vi "自动升级更新main.vi"() -> ()   [LabVIEW 2016, in "自动更新.lvlib"]
panel:
  out "waittime":u8
  out "有新版本":bool
  out "下载的文件名":string
  out "最新版本获取进度":u8(slide) scale=0.0..100.0
  # "版本获取中，请稍后！"
  # "s"
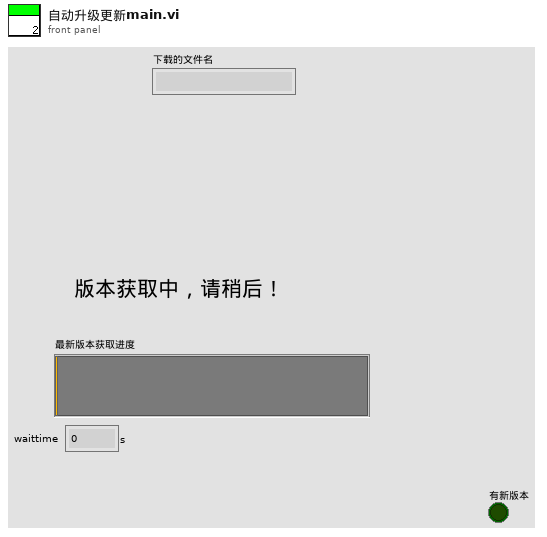
[diagram p1: front panel]
types:
  T1 = enum16{"get version information", "get success", "contact", "over"}
  T2 = cluster{"网络灯":bool, "接收中":bool, "已接收百分比":u8, "接收成功次数":dbl, "当前步骤":enum16{"init", "receivehead", "receivecontent", "receivesuccess", "over"}, "文件名":string, "error out":errorcluster}
  T3 = enum16{"open", "replace", "create", "open or create", "replace or create", "replace or create with confirmation"}
  T4 = enum32{"Bad", "Idle", "Run top level", "Running"}
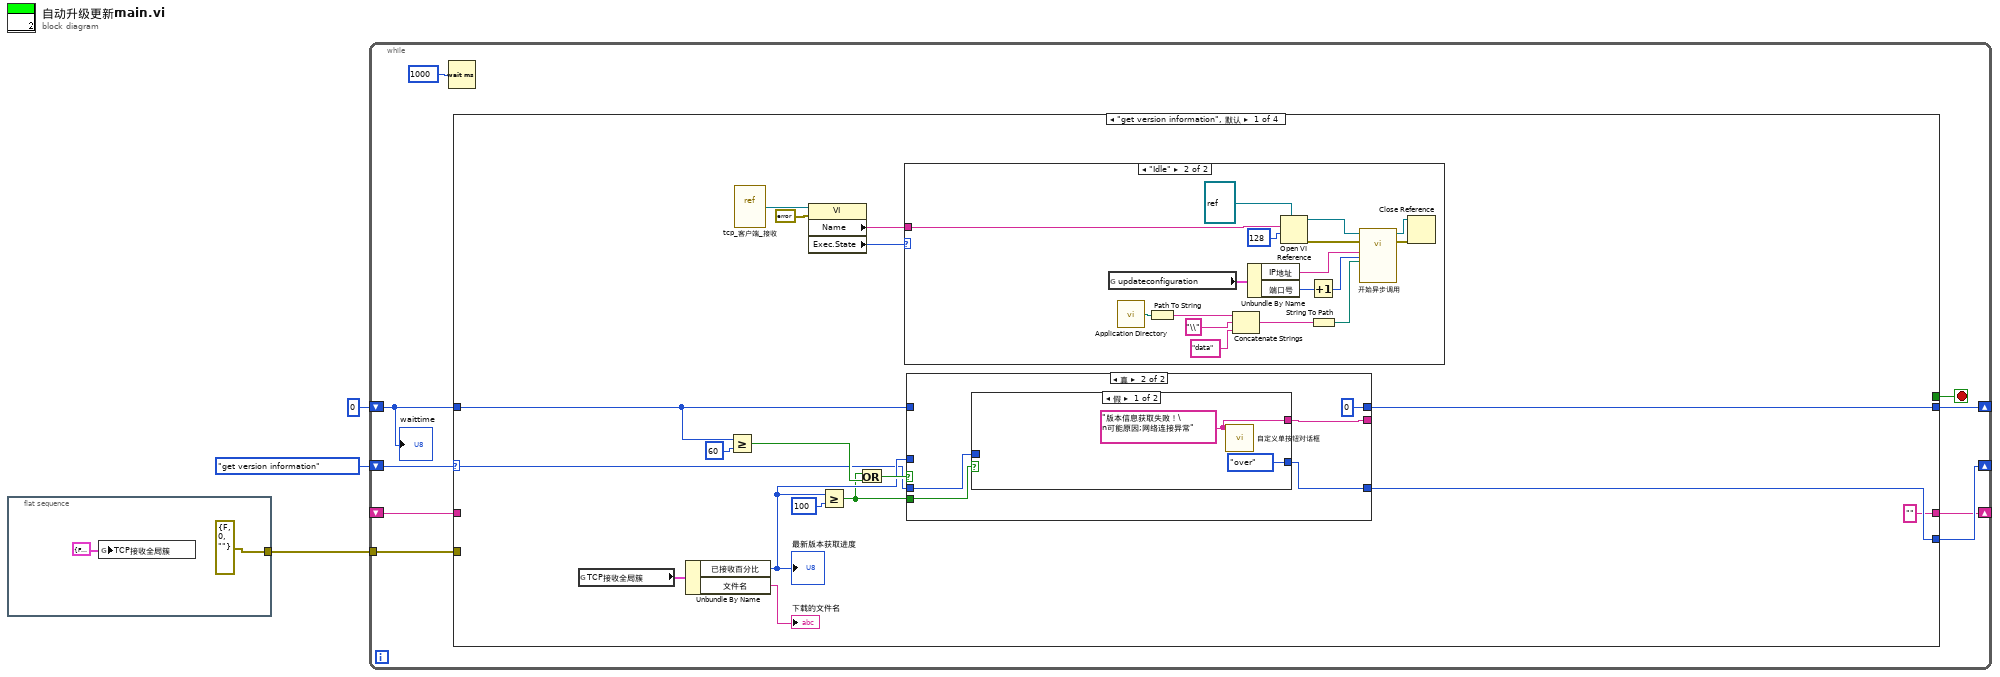
[diagram p0: block diagram]
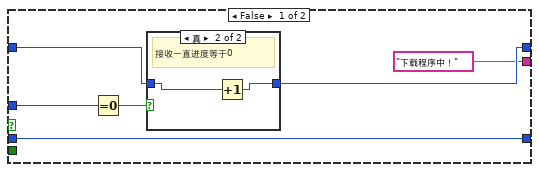
[diagram p2: hidden frame]
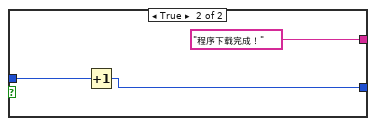
[diagram p4: hidden frame]
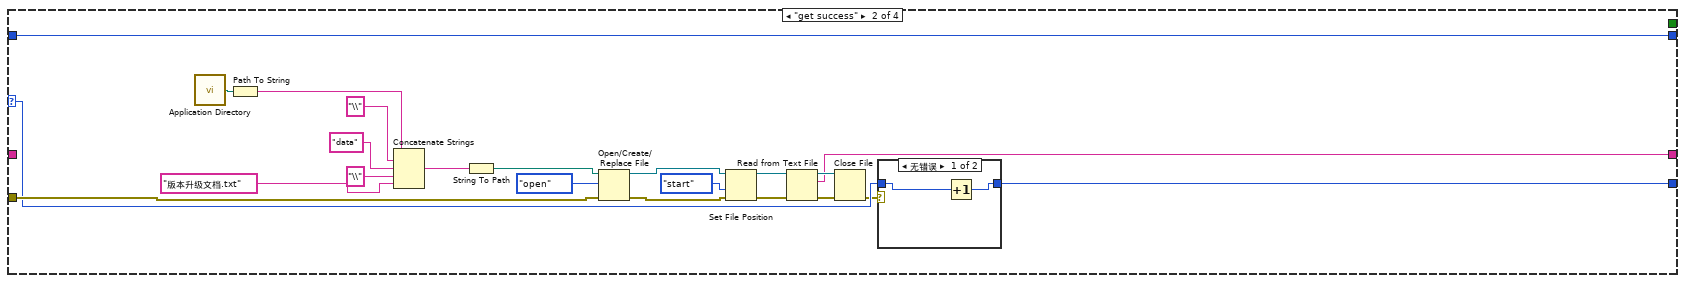
[diagram p6: hidden frame]
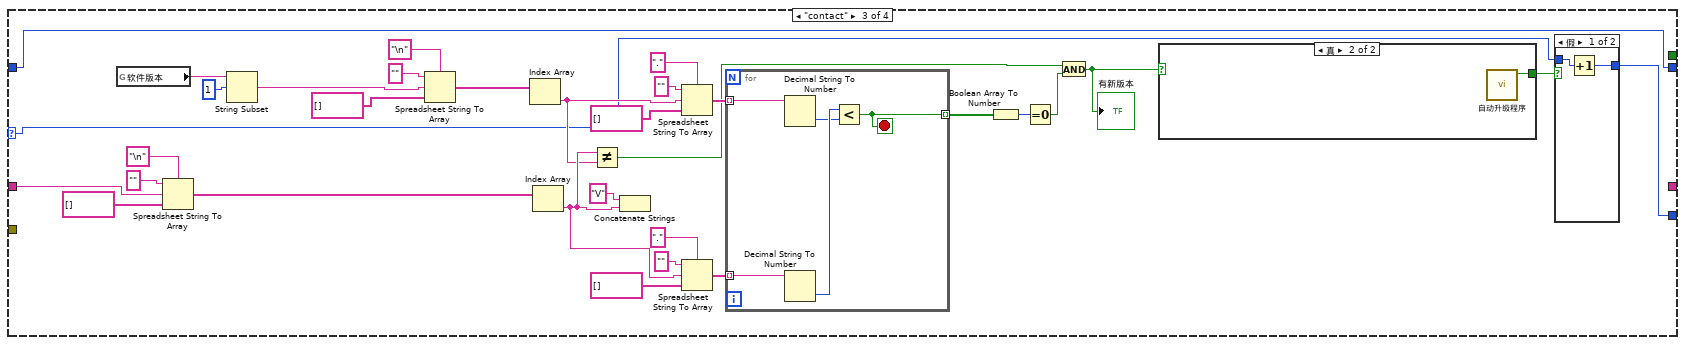
[diagram p8: hidden frame]
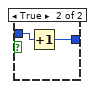
[diagram p9: hidden frame]
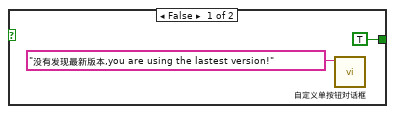
[diagram p10: hidden frame]
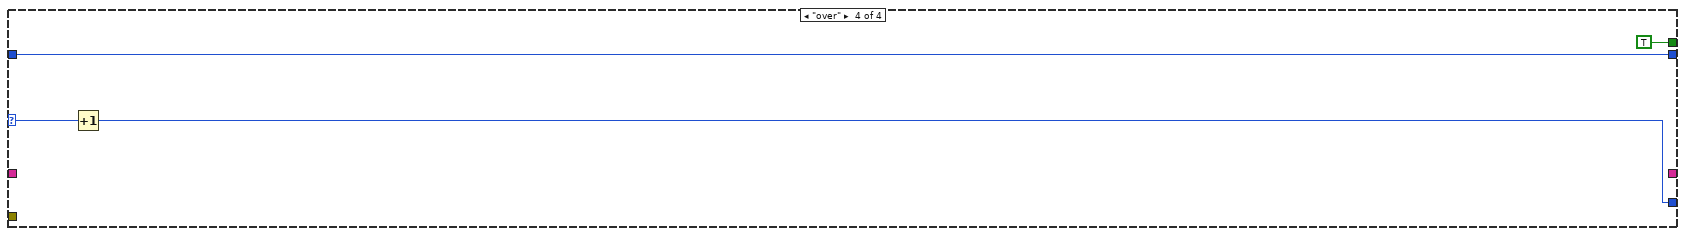
[diagram p11: hidden frame]
diagram:
  n1 = flat-sequence {
    tunnel: [errorcluster {"status"=FALSE, "code"=0, "source"=""} ("错误常量")] -> w1
    frame #0 {
      n2 = global write "全局变量1.vi" "TCP接收全局簇"(T2 {"网络灯"=FALSE, "接收中"=FALSE, "已接收百分比"=0, "接收成功次数"=0.0, "当前步骤"=enum."init", "文件名"="", "error out"={"status"=FALSE, "code"=0, "source"=""}} ("TCP接收全局簇")) -> ()
    }
  }
  n3 = while {
    shift-right: [w10] -> _
    shift-left: T1."get version information" -> [w13]
    shift-right: [w11] -> _
    shift-left: u8 0 ("y") -> [w12]
    tunnel: w1 -> [w9]
    shift-right: [w8] -> _
    shift-left: _ -> [w7]
    stop <- w6 stop-if-true
    n4 = Wait (ms)(milliseconds to wait=u32 1000 ("等待时间（毫秒）")) -> ()  [unwired: 1 out]
    n5 = case shown="\"get version information\", 默认" w13 {
      selector: w13 -> [w17 w76 w95 w138]
      tunnel: w12 -> [w19 w68 w93 w139]
      tunnel: [w18 w68 w93 w139] -> w11
      tunnel: [w16 w75 w94 w137] -> w10
      tunnel: w9 -> [_ w77 _ _]
      tunnel: ["" w69 _ _] -> w8
      tunnel: w7 -> [_ _ w98 _]
      tunnel: [_ _ _ TRUE] -> w6
      frame "get version information", Default {
        n6 = global read "全局变量1.vi" "TCP接收全局簇"() -> (w22:T2)
        n7 = Unbundle By Name(w22) -> ("已接收百分比"=w23:u8, "文件名"=→"下载的文件名":string)
        "最新版本获取进度" <- w23
        n8 = Greater Or Equal?(x=w19, y=u8 60) -> (x >= y?=w25:bool)
        n9 = vi-ref "tcp_客户端_接收.vi"() -> (w31:refnum<vi>)
        n10 = property class="VI"(reference=w31, error in=errorcluster {"status"=FALSE, "code"=0, "source"=""} ("错误输出")) -> ("Name"=w30:string, "Exec.State"=w28:T4)  [unwired: 2 out]
        n11 = Greater Or Equal?(x=w23, y=u8 100) -> (x >= y?=w21:bool)
        n12 = Or(x=w21, y=w25) -> (x .or. y?=w24:bool)
        n13 = case shown="\"Idle\"" w28 {
          tunnel: w30 -> [_ w67]
          frame "Bad", Default {
          }
          frame "Idle" {
            n14 = global read "update全局.vi" "updateconfiguration"() -> (w60:cluster{"IP地址":string, "端口号":i32})
            n15 = call <vilib>:"Application Directory.vi"() -> ("Application Directory"=w56:path)
            n16 = Path To String(path=w56) -> (string=w53:string)
            n17 = Concatenate Strings(w53, "\\" ("字符串"), "data" ("字符串")) -> (w57:string)
            n18 = Unbundle By Name(w60) -> ("IP地址"=w59:string, "端口号"=w58:i32)
            n19 = Open VI Reference(type specifier VI Refnum (for type only)=refnum<vi> refnum, vi path=w67, options=128 ("选项")) -> (vi reference=w65:refnum<vi>, error out=w63:errorcluster)  [unwired: 3 in]
            n20 = Increment(x=w58) -> (x+1=w51:i32)
            n21 = String To Path(string=w57) -> (path=w52:path)
            n22 = call-by-ref "开始异步调用"(reference=w65, error in=w63, "IP地址"=w59, "端口号"=w51, "储存路径"=w52) -> (reference out=w61:refnum<vi>, error out=w62:errorcluster)  [unwired: 17 in]
            n23 = Close Reference(reference=w61, error in (no error)=w62) -> ()  [unwired: 1 out]
          }
        }
        n24 = case shown="真" w24 {
          tunnel: w19 -> [w37 _]
          tunnel: [w36 u8 0] -> w18
          tunnel: w23 -> [w34 _]
          tunnel: [w33 w41] -> w16
          tunnel: w17 -> [w33 w42]
          tunnel: ["下载程序中！" w43] -> _
          tunnel: w21 -> [_ w44]
          frame False {
            n25 = Equal To 0?(x=w34) -> (x = 0?=w35:bool)
            n26 = case shown="真" w35 {
              tunnel: w37 -> [w38 w40]
              tunnel: [w38 w39] -> w36
              frame False {
              }
              frame True {
                # "接收一直进度等于0"
                n27 = Increment(x=w40) -> (x+1=w39:u8)
              }
            }
          }
          frame True {
            n28 = case shown="假" w44 {
              tunnel: [w47 "程序下载完成！"] -> w43
              tunnel: w42 -> [_ w49]
              tunnel: [T1."over" w48] -> w41
              frame False {
                w47 = "版本信息获取失败！\n可能原因;网络连接异常"
                n29 = call "自定义单按钮对话框.vi"("消息"=w47) -> ()  [unwired: 11 in]
              }
              frame True {
                n30 = Increment(x=w49) -> (x+1=w48:T1)
              }
            }
          }
        }
      }
      frame "get success" {
        n31 = call <vilib>:"Application Directory.vi"() -> ("Application Directory"=w82:path)
        n32 = Path To String(path=w82) -> (string=w85:string)
        n33 = Concatenate Strings(w85, "\\" ("字符串"), "data" ("字符串"), "\\" ("字符串"), "版本升级文档.txt" ("字符串")) -> (w79:string)
        n34 = String To Path(string=w79) -> (path=w78:path)
        n35 = Open/Create/Replace File(file path (use dialog)=w78, error in=w77, operation (0:open)=T3."open" ("操作(0:open)")) -> (refnum out=w88:refnum<file>, error out=w87:errorcluster)  [unwired: 3 in, 1 out]
        n36 = Set File Position(refnum=w88, from (0:start)=enum16{"start", "end", "current"}."start" ("自（0:起始）"), error in=w87) -> (refnum out=w73:refnum<file>, error out=w72:errorcluster)  [unwired: 1 in]
        n37 = Read from Text File(file (use dialog)=w73, error in=w72) -> (refnum out=w74:refnum<file>, text=w69:string, error out=w71:errorcluster)  [unwired: 2 in, 1 out]
        n38 = Close File(refnum=w74, error in=w71) -> (error out=w70:errorcluster)  [unwired: 1 out]
        n39 = case shown="无错误" w70 {
          tunnel: w76 -> [w91 w92]
          tunnel: [w90 w92] -> w75
          frame No Error {
            n40 = Increment(x=w91) -> (x+1=w90:T1)
          }
          frame Error {
          }
        }
      }
      frame "contact" {
        n41 = global read "update全局.vi" "软件版本"() -> (w116:string)
        n42 = Spreadsheet String To Array(delimiter (Tab)="\n" ("分隔符(Tab)"), format string="" ("格式字符串"), spreadsheet string=w98, array type (2D Dbl)=string[] []) -> (array=w120:string[])
        n43 = String Subset(string=w116, offset (0)=1 ("偏移量(0)")) -> (substring=w111:string)  [unwired: 1 in]
        n44 = Spreadsheet String To Array(delimiter (Tab)="\n" ("分隔符(Tab)"), format string="" ("格式字符串"), spreadsheet string=w111, array type (2D Dbl)=string[] []) -> (array=w110:string[])
        n45 = Index Array(array=w110) -> (element=w101:string)  [unwired: 1 in]
        n46 = Index Array(array=w120) -> (element=w102:string)  [unwired: 1 in]
        n47 = Not Equal?(x=w102, y=w101) -> (x != y?=w99:bool)
        n48 = Concatenate Strings("V" ("字符串"), w102) -> ()  [unwired: 1 out]
        n49 = Spreadsheet String To Array(delimiter (Tab)="." ("分隔符(Tab)"), format string="" ("格式字符串"), spreadsheet string=w101, array type (2D Dbl)=string[] []) -> (array=w105:string[])
        n50 = Spreadsheet String To Array(delimiter (Tab)="." ("分隔符(Tab)"), format string="" ("格式字符串"), spreadsheet string=w102, array type (2D Dbl)=string[] []) -> (array=w106:string[])
        n51 = for {
          tunnel: w106 -> [w134] mode=indexing
          tunnel: w105 -> [w136] mode=indexing
          tunnel: [w135] -> w104 mode=indexing
          stop <- w135 stop-if-true
          n52 = Decimal String To Number(string=w136) -> (number=w132:i32)  [unwired: 2 in, 1 out]
          n53 = Decimal String To Number(string=w134) -> (number=w133:i32)  [unwired: 2 in, 1 out]
          n54 = Less?(x=w133, y=w132) -> (x < y?=w135:bool)
        }
        n55 = Boolean Array To Number(Boolean array=w104) -> (number=w103:u32)
        n56 = Equal To 0?(x=w103) -> (x = 0?=w100:bool)
        n57 = And(x=w99, y=w100) -> (x .and. y?=w97:bool)
        "有新版本" <- w97
        n58 = case shown="真" w97 {
          tunnel: [TRUE ("确定") w131] -> w96
          frame False {
            n59 = call "自定义单按钮对话框.vi"("消息"="没有发现最新版本,you are using the lastest version!") -> ()  [unwired: 11 in]
          }
          frame True {
            n60 = call "自动升级程序.vi"() -> ("确定"=w131:bool)  [unwired: 10 in, 1 out]
          }
        }
        n61 = case shown="假" w96 {
          tunnel: w95 -> [w126 w128]
          tunnel: [w125 w127] -> w94
          frame False {
            n62 = Increment(x=w126) -> (x+1=w125:T1)
          }
          frame True {
            n63 = Increment(x=w128) -> (x+1=w127:T1)
          }
        }
      }
      frame "over" {
        n64 = Increment(x=w138) -> (x+1=w137:T1)
      }
    }
    "waittime" <- w12
  }
